vi "Kiwi_Get_Set_Refnum.vi"(8 "error in (no error)":errorcluster, 9 "menu":T10=enum."get", 10 "refnum name":string, 11 "Kiwi DevRef In":T1={"Motor A"={"DeviceStatus"={"status"=FALSE, "code"=0, "source"=""}, "Type"=enum."PWM", "PWM"={"PWM Channel"=enum."Invalid", "DeadBand"={"Name"="", "maxPositivePwm"=0, "minPositivePwm"=0, "centerPwm"=0, "maxNegativePwm"=0, "minNegativePwm"=0, "angularRange"=0}}, "CAN"={"Device Number"=0, "Control Mode"=enum."Percent VBus", "Semaphore"=refnum, "Max Vout"=12.0, "TalonSRX Control Mode"=enum."Percent VBus"}, "Invert"=FALSE}, "Motor B"={"DeviceStatus"={"status"=FALSE, "code"=0, "source"=""}, "Type"=enum."PWM", "PWM"={"PWM Channel"=enum."Invalid", "DeadBand"={"Name"="", "maxPositivePwm"=0, "minPositivePwm"=0, "centerPwm"=0, "maxNegativePwm"=0, "minNegativePwm"=0, "angularRange"=0}}, "CAN"={"Device Number"=0, "Control Mode"=enum."Percent VBus", "Semaphore"=refnum, "Max Vout"=12.0, "TalonSRX Control Mode"=enum."Percent VBus"}, "Invert"=FALSE}, "Motor C"={"DeviceStatus"={"status"=FALSE, "code"=0, "source"=""}, "Type"=enum."PWM", "PWM"={"PWM Channel"=enum."Invalid", "DeadBand"={"Name"="", "maxPositivePwm"=0, "minPositivePwm"=0, "centerPwm"=0, "maxNegativePwm"=0, "minNegativePwm"=0, "angularRange"=0}}, "CAN"={"Device Number"=0, "Control Mode"=enum."Percent VBus", "Semaphore"=refnum, "Max Vout"=12.0, "TalonSRX Control Mode"=enum."Percent VBus"}, "Invert"=FALSE}, "Config Consts"={"Arx"=0.0, "Ay"=0.0, "Brx"=0.0, "By"=0.0, "Cr"=0.0, "Cy"=0.0, "Cx"=0.0}, "status"={"status"=FALSE, "code"=0, "source"=""}}) -> (0 "error out":errorcluster, 2 "Kiwi DevRef Out":T1={"Motor A"={"DeviceStatus"={"status"=FALSE, "code"=0, "source"=""}, "Type"=enum."PWM", "PWM"={"PWM Channel"=enum."Invalid", "DeadBand"={"Name"="", "maxPositivePwm"=0, "minPositivePwm"=0, "centerPwm"=0, "maxNegativePwm"=0, "minNegativePwm"=0, "angularRange"=0}}, "CAN"={"Device Number"=0, "Control Mode"=enum."Percent VBus", "Semaphore"=refnum, "Max Vout"=12.0, "TalonSRX Control Mode"=enum."Percent VBus"}, "Invert"=FALSE}, "Motor B"={"DeviceStatus"={"status"=FALSE, "code"=0, "source"=""}, "Type"=enum."PWM", "PWM"={"PWM Channel"=enum."Invalid", "DeadBand"={"Name"="", "maxPositivePwm"=0, "minPositivePwm"=0, "centerPwm"=0, "maxNegativePwm"=0, "minNegativePwm"=0, "angularRange"=0}}, "CAN"={"Device Number"=0, "Control Mode"=enum."Percent VBus", "Semaphore"=refnum, "Max Vout"=12.0, "TalonSRX Control Mode"=enum."Percent VBus"}, "Invert"=FALSE}, "Motor C"={"DeviceStatus"={"status"=FALSE, "code"=0, "source"=""}, "Type"=enum."PWM", "PWM"={"PWM Channel"=enum."Invalid", "DeadBand"={"Name"="", "maxPositivePwm"=0, "minPositivePwm"=0, "centerPwm"=0, "maxNegativePwm"=0, "minNegativePwm"=0, "angularRange"=0}}, "CAN"={"Device Number"=0, "Control Mode"=enum."Percent VBus", "Semaphore"=refnum, "Max Vout"=12.0, "TalonSRX Control Mode"=enum."Percent VBus"}, "Invert"=FALSE}, "Config Consts"={"Arx"=0.0, "Ay"=0.0, "Brx"=0.0, "By"=0.0, "Cr"=0.0, "Cy"=0.0, "Cx"=0.0}, "status"={"status"=FALSE, "code"=0, "source"=""}}, 3 "refnum names":string[](array[string]))   [LabVIEW 2015]
uses:
  <vilib>/Rock Robotics/WPI/Utilities/Refnum Registry Operation.ctl
  <userlib>/836-Library/Drive/kiwi/Kiwi_Dev_Ref.ctl
  <vilib>/Rock Robotics/WPI/MotorControl/WPI_MotorControlDeviceRef.ctl
  <vilib>/Rock Robotics/WPI/MotorControl/WPI_MotorControlType.ctl
  <vilib>/Rock Robotics/SystemInterfaces/DIO/FPGA_DIOPWMChannel.ctl
  <vilib>/Rock Robotics/WPI/PWM/WPI_PWMDeadband.ctl
  <vilib>/Rock Robotics/WPI/CAN/Jaguar/SubVIs/WPI_CANJaguar_ControlMode.ctl
  <vilib>/Rock Robotics/WPI/CAN/TalonSRX/WPI_CANTalonSRX_APIControlMode.ctl
  <userlib>/836-Library/Drive/kiwi/Kiwi_Cal_Constants.ctl
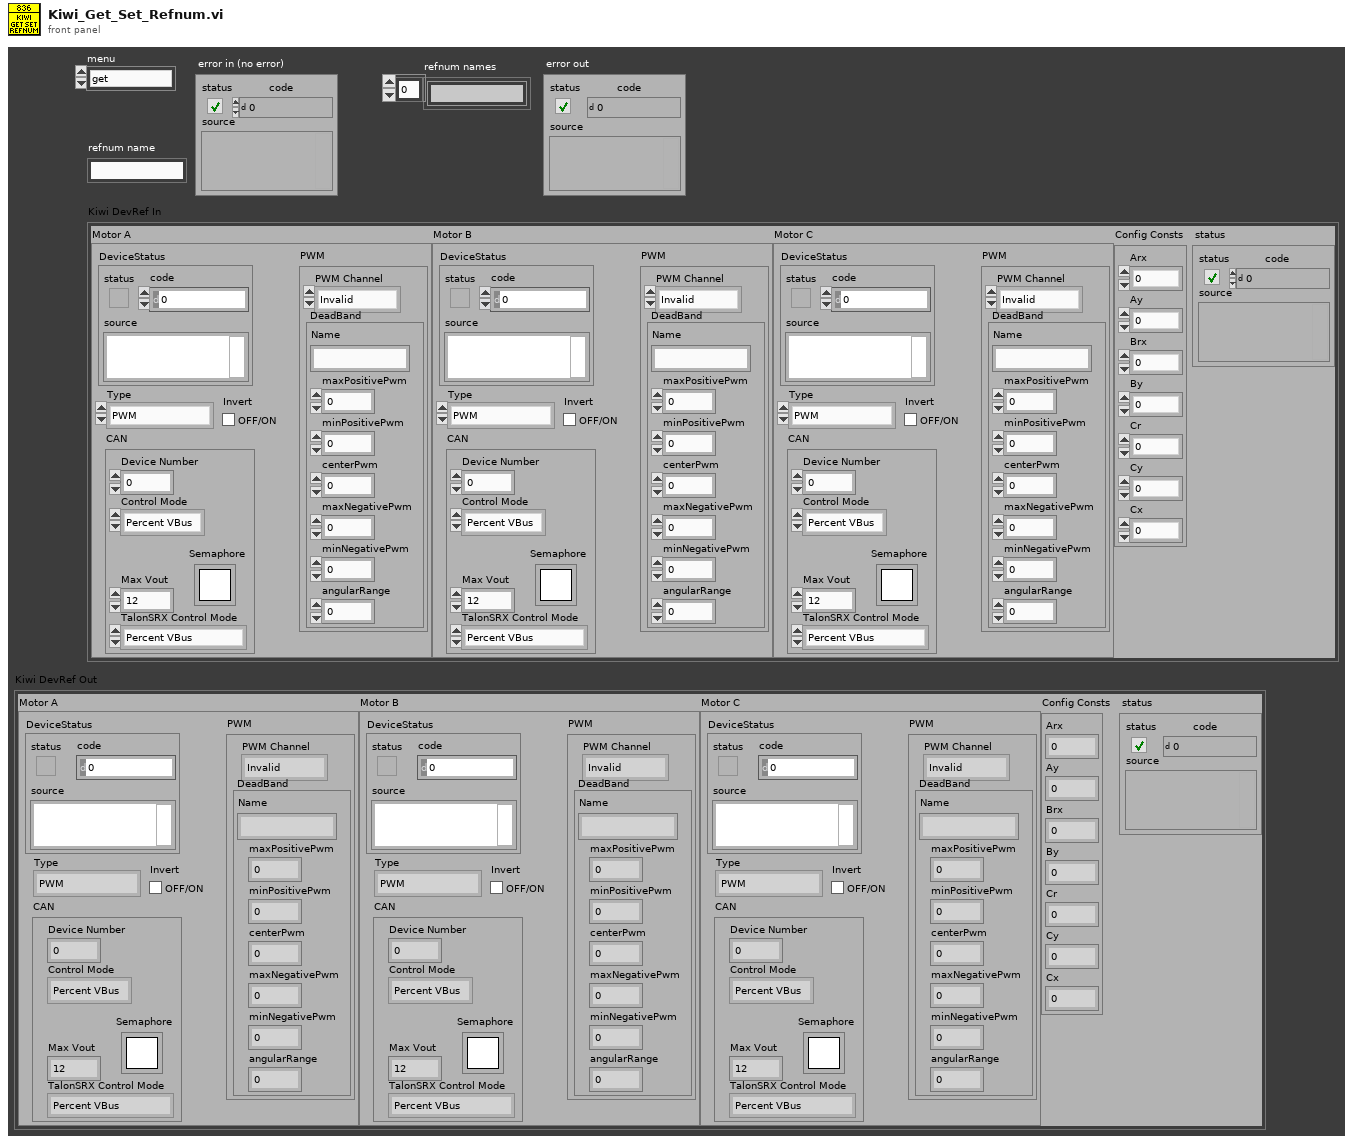
[diagram p1: front panel]
types:
  T1 = typedef "Kiwi_Dev_Ref.ctl" = cluster{"Motor A":T2, "Motor B":T2, "Motor C":T2, "Config Consts":T9, "status":errorcluster}
  T2 = typedef "WPI_MotorControlDeviceRef.ctl" = cluster{"DeviceStatus":errorcluster, "Type":T3, "PWM":cluster{"PWM Channel":T4, "DeadBand":T5}, "CAN":cluster{"Device Number":u8, "Control Mode":T6, "Semaphore":T7, "Max Vout":dbl, "TalonSRX Control Mode":T8}, "Invert":bool}
  T3 = typedef "WPI_MotorControlType.ctl" = enum16{"PWM", "CAN", "CANTalonSRX"}
  T4 = typedef "FPGA_DIOPWMChannel.ctl" = enum8{"PWM 0", "PWM 1", "PWM 2", "PWM 3", "PWM 4", "PWM 5", "PWM 6", "PWM 7", "PWM 8", "PWM 9", "PWM MXP 0", "PWM MXP 1", "PWM MXP 2", "PWM MXP 3", "PWM MXP 4", "PWM MXP 5", "PWM MXP 6", "PWM MXP 7", "PWM MXP 8", "PWM MXP 9", "Invalid"}
  T5 = typedef "WPI_PWMDeadband.ctl" = cluster{"Name":string, "maxPositivePwm":i32, "minPositivePwm":i32, "centerPwm":i32, "maxNegativePwm":i32, "minNegativePwm":i32, "angularRange":u16}
  T6 = typedef "WPI_CANJaguar_ControlMode.ctl" = enum8{"Percent VBus", "Current", "Speed", "Position", "Voltage"}
  T7 = typedef "Semaphore RefNum" = refnum<k1>
  T8 = typedef "WPI_CANTalonSRX_APIControlMode.ctl" = enum8{"Percent VBus", "Speed", "Position", "Slave", "Unchanged / Invalid", "Voltage Compensation", "Current", "Motion Profile"}
  T9 = typedef "Kiwi_Cal_Constants.ctl" = cluster{"Arx":dbl, "Ay":dbl, "Brx":dbl, "By":dbl, "Cr":dbl, "Cy":dbl, "Cx":dbl}
  T10 = typedef "Refnum Registry Operation.ctl" = enum16{"set", "get", "delete", "get all names", "read name"}
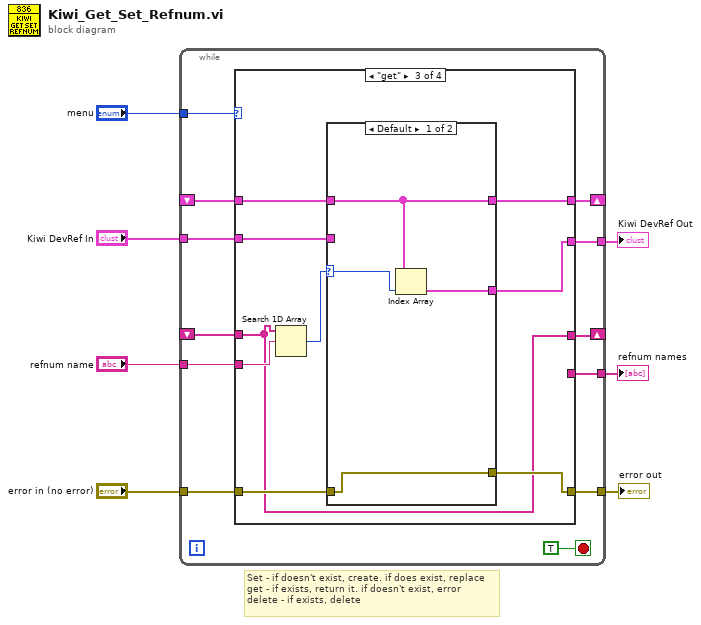
[diagram p0: block diagram]
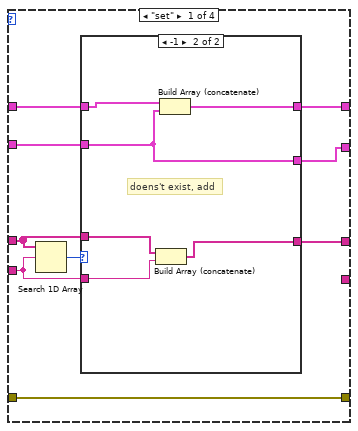
[diagram p2: hidden frame]
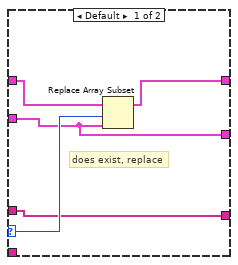
[diagram p3: hidden frame]
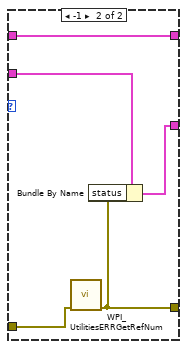
[diagram p5: hidden frame]
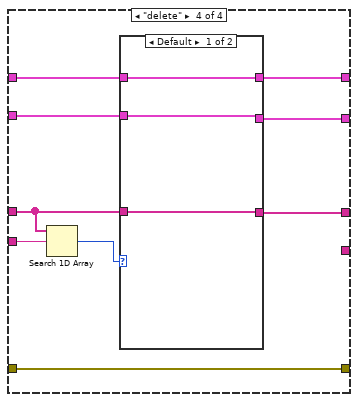
[diagram p6: hidden frame]
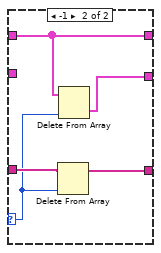
[diagram p7: hidden frame]
diagram:
  # "Set - if doesn't exist, create. if does exist, replace\nget - if exists, return it. if doesn't exist, error\ndelete - if exists, delete"
  n1 = while {
    tunnel: "menu" -> [w18]
    tunnel: "Kiwi DevRef In" -> [w17]
    tunnel: "refnum name" -> [w16]
    tunnel: "error in (no error)" -> [w15]
    shift-right: [w10] -> _
    shift-left: _ -> [w14]
    shift-right: [w13] -> _
    shift-left: _ -> [w12]
    tunnel: [w11] -> w3
    tunnel: [w9] -> w2
    tunnel: [w8] -> w1
    stop <- TRUE stop-if-true
    n2 = case shown="\"get\"" w18 {
      tunnel: w17 -> [w22 w42 w46 w68]
      tunnel: w16 -> [w25 _ w52 w70]
      tunnel: w15 -> [w28 w40 w47 w62]
      tunnel: w14 -> [w26 w41 w44 w64]
      tunnel: [w21 w43 w48 w66] -> w13
      tunnel: w12 -> [w23 w43 w50 w67]
      tunnel: [w20 w42 w49 w65] -> w11
      tunnel: [w24 w41 w44 w63] -> w10
      tunnel: [_ w41 _ _] -> w9
      tunnel: [w28 w40 w45 w62] -> w8
      frame "set" {
        n3 = Search 1D Array(1D array=w26, element=w25) -> (index of element=w27:i32)  [unwired: 1 in]
        n4 = case shown="-1" w27 {
          selector: w27 -> [w32 _]
          tunnel: w26 -> [w30 w39]
          tunnel: w25 -> [_ w38]
          tunnel: [w30 w37] -> w24
          tunnel: w23 -> [w33 w36]
          tunnel: w22 -> [w29 w34]
          tunnel: [w31 w35] -> w21
          tunnel: [w29 w34] -> w20
          frame Default {
            # "does exist, replace"
            n5 = Replace Array Subset(array=w33, new element=w29, index=w32) -> (w31:T1[])
          }
          frame -1 {
            # "doens't exist, add"
            n6 = Build Array (concatenate)(w39, w38) -> (w37:string[])
            n7 = Build Array (concatenate)(w36, w34) -> (w35:T1[])
          }
        }
      }
      frame "get all names", Default {
      }
      frame "get" {
        n8 = Search 1D Array(1D array=w44, element=w52) -> (index of element=w51:i32)  [unwired: 1 in]
        n9 = case shown="Default" w51 {
          selector: w51 -> [w56 _]
          tunnel: w50 -> [w54 w61]
          tunnel: [w55 w58] -> w49
          tunnel: [w54 w61] -> w48
          tunnel: w47 -> [w53 w60]
          tunnel: w46 -> [_ w59]
          tunnel: [w53 w57] -> w45
          frame Default {
            n10 = Index Array(array=w54, index=w56) -> (element=w55:T1)
          }
          frame -1 {
            n11 = call <vilib>:"WPI_UtilitiesERRGetRefNum.vi"("error in (no error)"=w60) -> ("ERRGetRefNum"=w57:errorcluster)  [unwired: 10 out]
            n12 = Bundle By Name(cluster=w59, "status"=w57) -> (w58:T1)
          }
        }
      }
      frame "delete" {
        n13 = Search 1D Array(1D array=w64, element=w70) -> (index of element=w69:i32)  [unwired: 1 in]
        n14 = case shown="Default" w69 {
          selector: w69 -> [_ w77]
          tunnel: [w72 w75] -> w65
          tunnel: w68 -> [w72 _]
          tunnel: w67 -> [w73 w76]
          tunnel: [w73 w76] -> w66
          tunnel: w64 -> [w71 w78]
          tunnel: [w71 w74] -> w63
          frame Default {
          }
          frame -1 {
            n15 = Delete From Array(array=w78, index=w77) -> (array with subset deleted=w74:string[])  [unwired: 1 in, 1 out]
            n16 = Delete From Array(array=w76, index=w77) -> (deleted portion=w75:T1)  [unwired: 1 in, 1 out]
          }
        }
      }
    }
  }
  "Kiwi DevRef Out" <- w3
  "error out" <- w1
  "refnum names" <- w2
